vi "NIIE_ni.com_iconlibrary.vi"(8 "error in (no error)":errorcluster {"code" min=0 max=0}) -> (0 "error out":errorcluster {"code" min=0 max=0})   [LabVIEW 2021]
doc: "<p>Select <strong>Tools<span class=\"U+187\">>></span>Synchronize with ni.com Icon Library</strong> from the <a href=\"nihelplauncher://docs/csh?context=lvcore_lvdialog_icon_editor\">Icon Editor</a> dialog box to display this dialog box.</p>\n<p>Use this dialog box to synchronize the <span class=\"Monospace\">LabVIEW Data\\Glyphs</span> directory with the most recent glyphs in the <a href=\"https://www.ni.com/r/expnr7\">Icon Library</a> at <span class=\"Monospace\">ni.com</span>.</p>\n<p>This dialog box includes the following components:</p>"
uses:
  MB CORE/TypeDefs/Array_Glyph List.ctl
  MB CORE/TypeDefs/Cluster_Glyph Data.ctl
  vi.lib/LabVIEW Icon API/lv_icon/Controls/Pathes.ctl
  lv_IconEditor.lvlib
  vi.lib/LabVIEW Icon API/lv_icon/lv_icon.lvlib
panel:
  in  "Array":T1(array[cluster])
  in  "Message in":string="Downloading files..."
  in  "Abort Button Text (\"\")":string="Cancel"
  in  "FP.Title":string="Downloading Icon Library Files"
  out "Icon Library":string="Icon Library"
  in  "Select / Deselect":bool
  in  "?":T2 {"Rectangle"."left" min=0 max=0; "Rectangle"."top" min=0 max=0; "Rectangle"."right" min=0 max=0; "Rectangle"."bottom" min=0 max=0}
  out "Install":string="Install"
  out "Glyph name":string="Name"
  out "SubFolder":string="Subfolder"
  out "Current Glyph":string="Current"
  in  "Glyph list":T3=[{"Install"=FALSE, "Current"=bytes[272], "Icon Library"=bytes[272], "Subfolder"="", "Name"=""}]
  in  "Help":bool
  in  "Cancel":bool
  in  "OK":bool
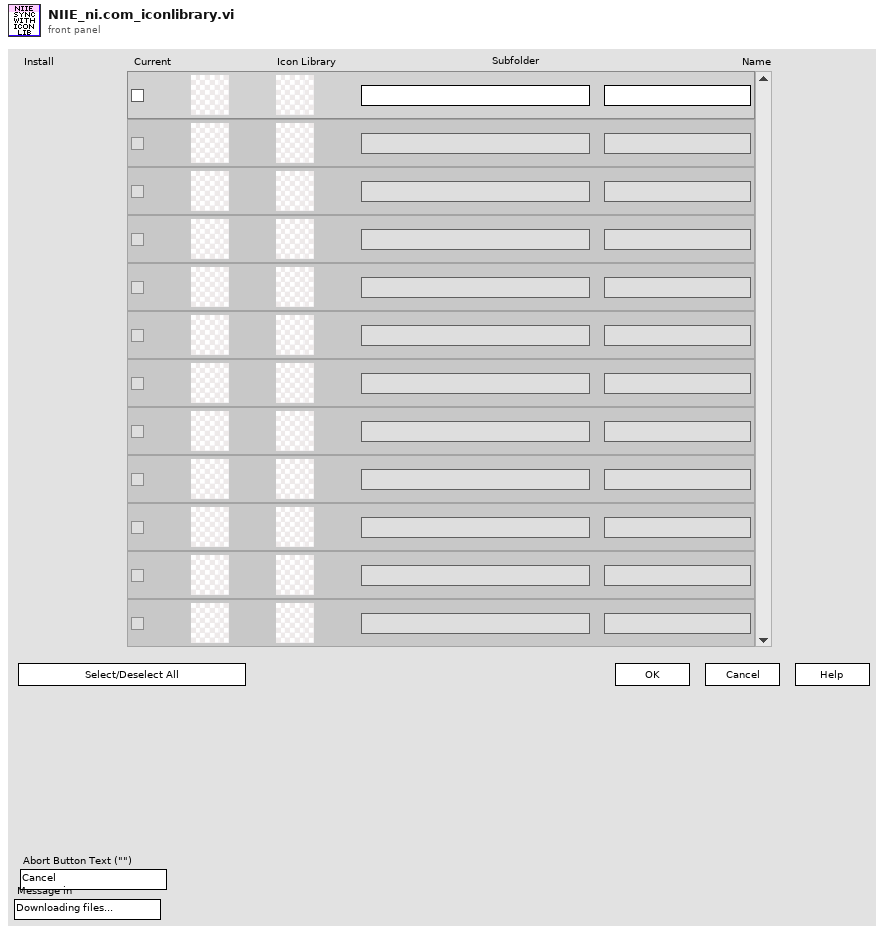
[diagram p1: front panel]
types:
  T1 = cluster{"Group folder":string, "FileName":string, "Rectangle":cluster{"left":i16, "top":i16, "right":i16, "bottom":i16}, "Path":path, "Image":picture}[]
  T2 = cluster{"Group folder":string, "FileName":string, "Rectangle":cluster{"left":i16, "top":i16, "right":i16, "bottom":i16}, "Path":path, "Image":picture}
  T3 = typedef "Array_Glyph List.ctl" = T4[]
  T4 = typedef "Cluster_Glyph Data.ctl" = cluster{"Install":bool, "Current":picture, "Icon Library":picture, "Subfolder":string, "Name":string}
  T5 = typedef "XMLDataStructureIconLibrary.ctl" = cluster{"imgExt":string, "glyphNameLoc":string, "glyphName":string, "type":string, "loctype":string, "imgName":string}
  T6 = typedef "Pathes.ctl" = enum16{"Root Path", "Icon Templates", "Icon Templates VI", "Icon Templates Lib", "Glyphs"}
  T7 = cluster{"File in zip file":string, "File name on disk":string, "Group":string}[]
  T8 = typedef "imagedata.ctl" = cluster{"image type":i32, "image depth":i32, "image":u8[], "mask":u8[], "colors":u32[], "Rectangle":cluster{"left":i16, "top":i16, "right":i16, "bottom":i16}}
  T9 = typedef "Cluster_Path&Icon.ctl" = cluster{"Rectangle":cluster{"left":i16, "top":i16, "right":i16, "bottom":i16}, "Path":path, "Image":picture, "Filter":string, "FileName":string}
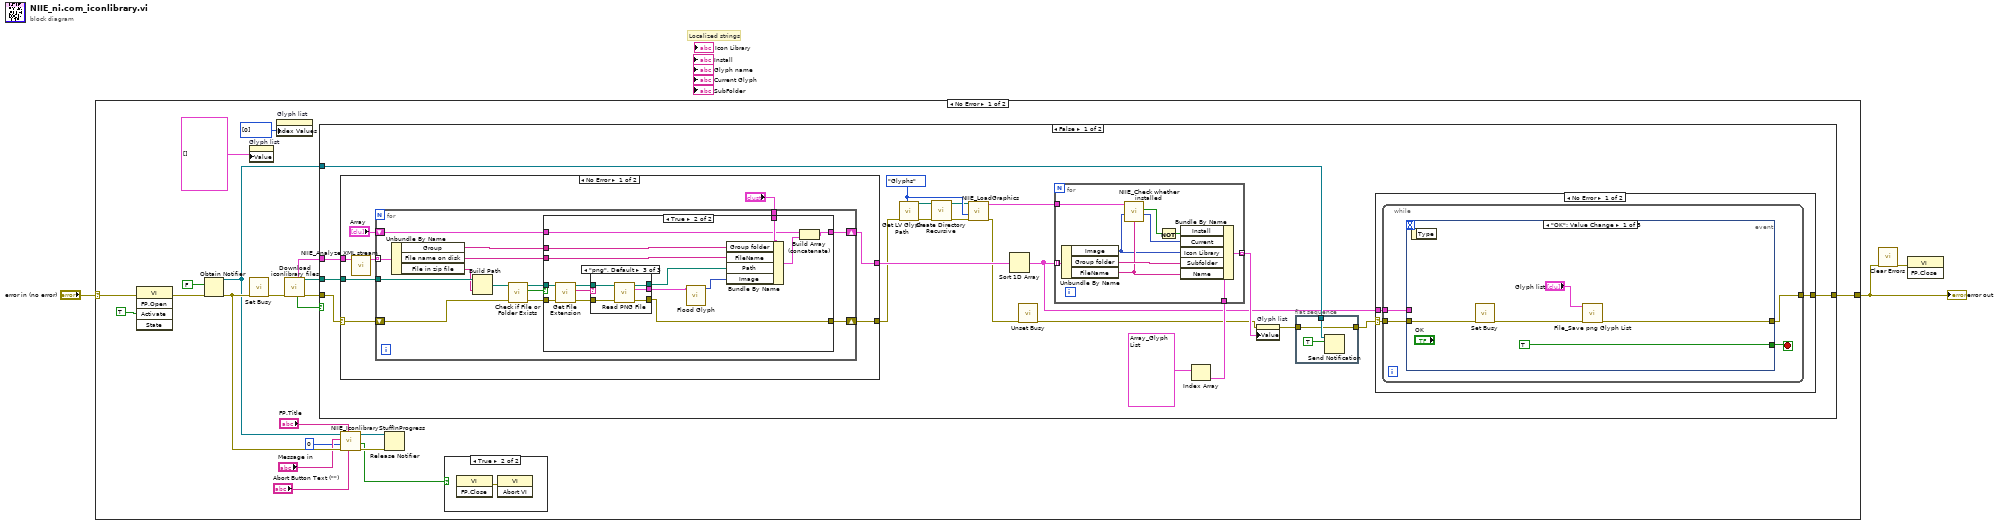
[diagram p0: block diagram]
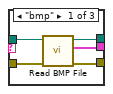
[diagram p4: hidden frame]
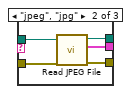
[diagram p5: hidden frame]
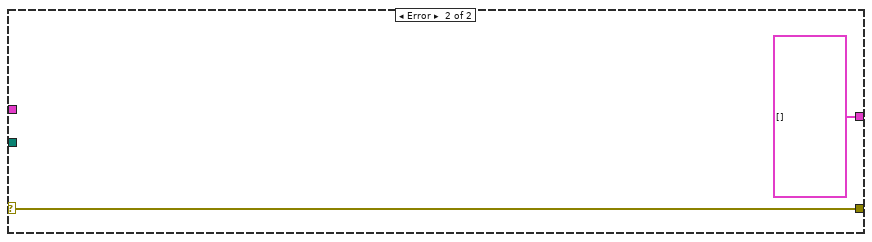
[diagram p6: hidden frame]
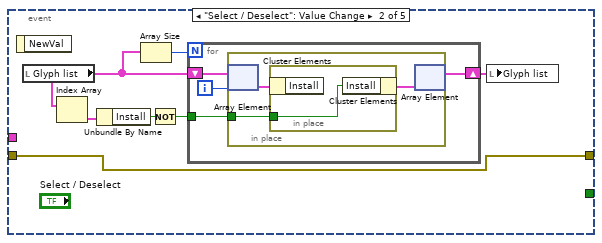
[diagram p7: hidden frame]
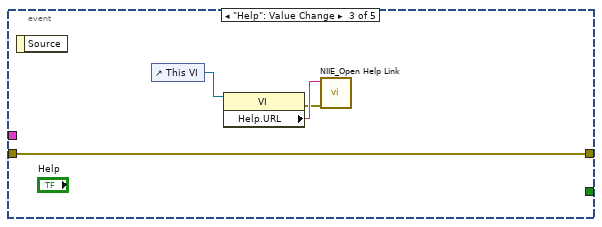
[diagram p8: hidden frame]
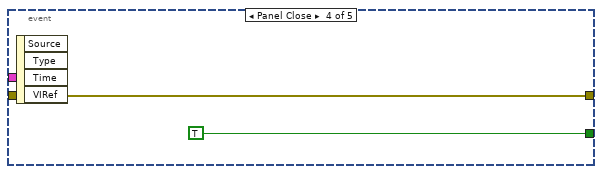
[diagram p9: hidden frame]
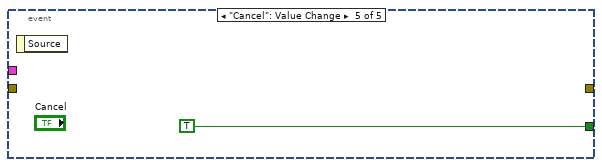
[diagram p10: hidden frame]
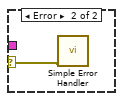
[diagram p11: hidden frame]
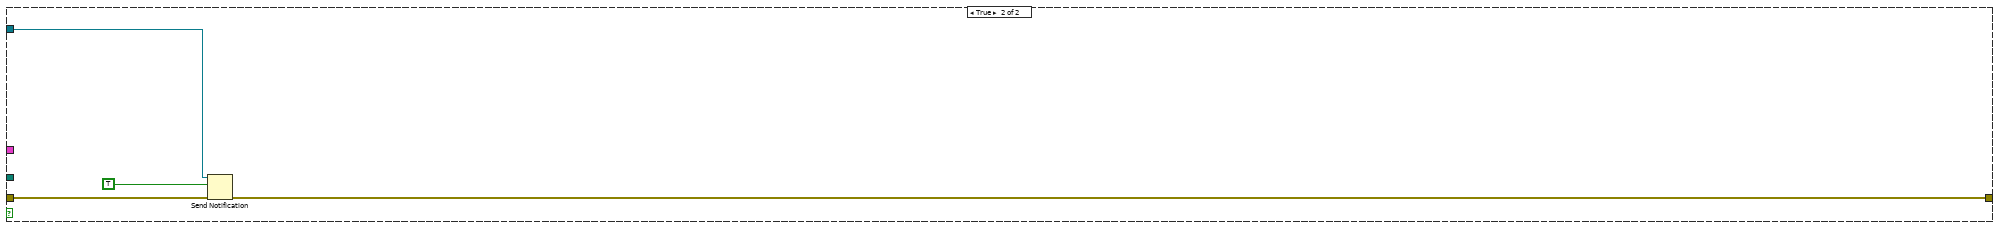
[diagram p12: hidden frame]
diagram:
  # "Localized strings"
  n1 = case shown="No Error" "error in (no error)" {
    selector: "error in (no error)" -> [w4 w155]
    tunnel: [w22 w155] -> w1
    frame No Error {
      n2 = invoke class="VI" method="FP.Open"(error in=w4, "Activate"=TRUE ("Activate?")) -> (error out=w6:errorcluster)  [unwired: 3 in, 4 out]
      n3 = Obtain Notifier(notification data type=FALSE, error in (no error)=w6) -> (notifier out=w9:refnum<notifier>, error out=w12:errorcluster)  [unwired: 2 in, 1 out]
      n4 = call <vilib>:"Set Busy.vi"("error in (no error)"=w12) -> ("error out"=w21:errorcluster)  [unwired: 3 in, 7 out]
      n5 = property on="Glyph list" class="Arr (strict)"("Value"=T3 [] ("Glyph list")) -> ()  [unwired: 2 in, 2 out]
      n6 = property on="Glyph list" class="Arr (strict)"("Index Values"=u32[] [0]) -> ()  [unwired: 2 in, 2 out]
      n7 = call "Download iconlibrary files.vi"("error in"=w21) -> ("error out"=w19:errorcluster, "parent path"=w23:path, "Cancelled?"=w17:bool, "XML Data"=w24:T5[])  [unwired: 7 out]
      n8 = case shown="False" w17 {
        tunnel: w24 -> [w46 _]
        tunnel: w23 -> [w45 _]
        tunnel: [w44 w151] -> w22
        tunnel: w19 -> [w34 w153]
        tunnel: w9 -> [w37 w152]
        frame False {
          w41 = Pathes."Glyphs" ("Path")
          n9 = case shown="No Error" w34 {
            selector: w34 -> [w49 w102]
            tunnel: w46 -> [w54 _]
            tunnel: [w48 T1 []] -> w33
            tunnel: w45 -> [w52 _]
            tunnel: [w51 w102] -> w31
            frame No Error {
              n10 = call "NIIE_Analyze XML stream.vi"("XML Data"=w54) -> ("Data"=w53:T7)  [unwired: 10 out]
              n11 = for {
                tunnel: w52 -> [w67]
                tunnel: w53 -> [w68] mode=indexing
                tunnel: "?" -> [w64]
                shift-right: [w55] -> w51
                shift-left: w49 -> [w58]
                shift-right: [w62] -> w48
                shift-left: "Array" -> [w61]
                n12 = Unbundle By Name(w68) -> ("Group"=w65:string, "File name on disk"=w63:string, "File in zip file"=w66:string)
                n13 = Build Path(base path=w67, name or relative path=w66) -> (appended path=w60:path)
                n14 = call <vilib>:"Check if File or Folder Exists.vi"("error in (no error)"=w58, "path"=w60) -> ("error out"=w56:errorcluster, "file or folder exists?"=w57:bool, "dup path"=w59:path)  [unwired: 7 in]
                n15 = case shown="True" w57 {
                  tunnel: w59 -> [_ w85]
                  tunnel: w56 -> [w69 w84]
                  tunnel: w65 -> [_ w79]
                  tunnel: w64 -> [_ w78]
                  tunnel: w63 -> [_ w77]
                  tunnel: [w70 w73] -> w62
                  tunnel: w61 -> [w70 w72]
                  tunnel: [w69 w71] -> w55
                  frame False {
                  }
                  frame True {
                    n16 = call <vilib>:"Get File Extension.vi"("error in (no error)"=w84, "file"=w85) -> ("error out"=w81:errorcluster, "lowercase file extension"=w82:string, "dup file"=w83:path)  [unwired: 7 out]
                    n17 = case shown="\"png\", Default" w82 {
                      tunnel: w83 -> [w89 w94 w100]
                      tunnel: w81 -> [w90 w95 w99]
                      tunnel: [w87 w93 w97] -> w76
                      tunnel: [w88 w92 w98] -> w80
                      tunnel: [w86 w91 w96] -> w71
                      frame "bmp" {
                        n18 = call <vilib>:"Read BMP File.vi"("error in (no error)"=w90, "path to BMP file"=w89) -> ("error out"=w86:errorcluster, "image data"=w87:T8, "path"=w88:path)  [unwired: 7 out]
                      }
                      frame "jpeg", "jpg" {
                        n19 = call <vilib>:"Read JPEG File.vi"("error in (no error)"=w95, "path to JPEG file"=w94) -> ("error out"=w91:errorcluster, "image data"=w93:T8, "path"=w92:path)  [unwired: 1 in, 6 out]
                      }
                      frame "png", Default {
                        n20 = call <vilib>:"Read PNG File.vi"("error in (no error)"=w99, "path to PNG file"=w100) -> ("error out"=w96:errorcluster, "image data"=w97:T8, "path"=w98:path)  [unwired: 1 in, 6 out]
                      }
                    }
                    n21 = call "Flood Glyph.vi"("Image Data"=w76) -> ("Pic Out"=w75:picture)  [unwired: 1 in, 9 out]
                    n22 = Bundle By Name(cluster=w78, "Group folder"=w79, "FileName"=w77, "Path"=w80, "Image"=w75) -> (w74:T2)
                    n23 = Build Array (concatenate)(w72, w74) -> (w73:T1)
                  }
                }
              }
            }
            frame Error {
            }
          }
          n24 = call "Get LV Glyph Path.vi"("Path"=w41, "error in (no error)"=w31) -> ("error out"=w30:errorcluster, "Requested Path"=w29:path)  [unwired: 1 in, 7 out]
          n25 = call <vilib>:"Create Directory Recursive.vi"("error in (no error)"=w30, "directory"=w29) -> ("error out"=w27:errorcluster, "directory copy"=w28:path)  [unwired: 1 in, 3 out]
          n26 = call "NIIE_LoadGraphics.vi"("Error"=w27, "Source"=w41, "Graphic Root Folder"=w28) -> ("Error Out"=w26:errorcluster, "Glyphs Out"=w40:T9[])  [unwired: 3 in, 4 out]
          n27 = Sort 1D Array(array=w33) -> (sorted array=w32:T1)
          n28 = call <vilib>:"Unset Busy.vi"("error in (no error)"=w26) -> ("error out"=w38:errorcluster)  [unwired: 1 in, 9 out]
          n29 = Index Array(array=T3 [{"Install"=FALSE, "Current"=bytes[272], "Icon Library"=bytes[272], "Subfolder"="", "Name"=""}] ("Cluster")) -> (element=w43:T4)  [unwired: 1 in]
          n30 = for {
            tunnel: w32 -> [w149] mode=indexing
            tunnel: w43 -> [w150]
            tunnel: w40 -> [w147]
            tunnel: [w146] -> w39 mode=indexing
            n31 = Unbundle By Name(w149) -> ("Image"=w141:picture, "Group folder"=w148:string, "FileName"=w142:string)
            n32 = call "NIIE_Check whether installed.vi"("Glyph Name"=w142, "Glyph Pic"=w141, "Glyphs[]"=w147) -> ("Image Out"=w143:picture, "Match? Out"=w145:bool)  [unwired: 1 in, 6 out]
            n33 = Not(x=w145) -> (.not. x?=w144:bool)
            n34 = Bundle By Name(cluster=w150, "Install"=w144, "Current"=w143, "Icon Library"=w141, "Subfolder"=w148, "Name"=w142) -> (w146:T4)
          }
          n35 = property on="Glyph list" class="Arr (strict)"(error in=w38, "Value"=w39) -> (error out=w36:errorcluster)  [unwired: 1 in, 1 out]
          n36 = flat-sequence {
            tunnel: w37 -> [w105]
            tunnel: w36 -> [w103]
            tunnel: [w103] -> w35
            frame #0 {
              n37 = Send Notification(notification=TRUE, notifier=w105) -> ()  [unwired: 1 in, 2 out]
            }
          }
          n38 = case shown="No Error" w35 {
            selector: w35 -> [w106 w140]
            tunnel: w32 -> [w108 _]
            tunnel: [w107 _] -> w44
            frame No Error {
              n39 = while {
                tunnel: w106 -> [w112]
                tunnel: w108 -> [w110]
                tunnel: [w109] -> w107
                stop <- w111 stop-if-true
                n40 = event shown="[0] \"OK\": Value Change" {
                  selector: _ -> [_ _ _ _ _]
                  dyn-events: _ -> [_ _ _ _ _]
                  timeout: _ -> [_ _ _ _ _]
                  tunnel: w112 -> [w115 w120 w136 w137 _]
                  tunnel: [TRUE _ _ TRUE TRUE] -> w111
                  tunnel: [w113 w120 w136 w137 _] -> w109
                  tunnel: w110 -> [_ _ _ _ _]
                  event "OK": Value Change {
                    n41 = event-data() -> ()  [unwired: 1 in, 1 out]
                    n42 = call <vilib>:"Set Busy.vi"("error in (no error)"=w115) -> ("error out"=w114:errorcluster)  [unwired: 3 in, 7 out]
                    n43 = call "File_Save png Glyph List.vi"("error in (no error)"=w114, "Glyph list"="Glyph list") -> ("error out"=w113:errorcluster)  [unwired: 9 out]
                  }
                  event "Select / Deselect": Value Change {
                    n44 = event-data() -> ()  [unwired: 1 in, 1 out]
                    n45 = local read "Glyph list"() -> (w118:T3)
                    n46 = Index Array(array=w118) -> (element=w124:T4)  [unwired: 1 in]
                    n47 = Unbundle By Name(w124) -> ("Install"=w123:bool)
                    n48 = Array Size(array=w118) -> (size(s)=w119:i32)
                    n49 = Not(x=w123) -> (.not. x?=w122:bool)
                    n50 = for {
                      N: w119 -> [_]
                      shift-right: [w125] -> w121
                      shift-left: w118 -> [w128]
                      tunnel: w122 -> [w126]
                      i -> [w127]
                      n51 = in-place {
                        in-place-border: w126 -> [w130]
                        n52 = in-place-array #1(w128, w127) -> (w131:T4)
                        n53 = in-place {
                          in-place-border: w130 -> [w132]
                          n54 = in-place-cluster #2(w131) -> ()  [unwired: 1 out]
                          n55 = in-place-cluster #2("Install"=w132) -> (w129:T4)
                        }
                        n56 = in-place-array #1(w129) -> (w125:T3)  [unwired: 1 out]
                      }
                    }
                    n57 = local write "Glyph list"(w121) -> ()
                  }
                  event "Help": Value Change {
                    n58 = event-data() -> ()  [unwired: 1 in, 1 out]
                    n59 = control-ref of="This VI"() -> (w135:refnum<vi>)
                    n60 = property class="VI"(reference=w135) -> (error out=w133:errorcluster, "Help.URL"=w134:string)  [unwired: 1 in, 1 out]
                    n61 = call "NIIE_Open Help Link.vi"("error in (no error)"=w133, "Help.URL"=w134) -> ()  [unwired: 9 in, 1 out]
                  }
                  event Panel Close {
                    n62 = event-data() -> ()  [unwired: 1 in, 4 out]
                  }
                  event "Cancel": Value Change {
                    n63 = event-data() -> ()  [unwired: 1 in, 1 out]
                  }
                }
              }
            }
            frame Error {
              n64 = call <vilib>:"Simple Error Handler.vi"("error in (no error)"=w140) -> ()  [unwired: 3 in, 6 out]
            }
          }
        }
        frame True {
          n65 = Send Notification(notification=TRUE, notifier=w152, error in (no error)=w153) -> (error out=w151:errorcluster)  [unwired: 1 out]
        }
      }
      n66 = call "NIIE_IconlibraryStuffInProgress.vi"("Abort Button Text (\"\")"="Abort Button Text (\"\")", "FP.Title"="FP.Title", "error in (no error)"=w12, "Show FP Timeout (ms)"=0, "Message in"="Message in", "Close Notifier"=w9) -> ("error out"=w15:errorcluster, "Aborted"=w10:bool, "Close Notifier out"=w14:refnum<notifier>)  [unwired: 3 in]
      n67 = Release Notifier(notifier=w14, error in (no error)=w15) -> ()  [unwired: 1 in, 3 out]
      n68 = case shown="True" w10 {
        frame False {
        }
        frame True {
          n69 = invoke class="VI" method="FP.Close"() -> (error out=w25:errorcluster)  [unwired: 3 in, 2 out]
          n70 = invoke class="VI" method="Abort VI"(error in=w25) -> ()  [unwired: 2 in, 3 out]
        }
      }
    }
    frame Error {
    }
  }
  "error out" <- w1
  n71 = call <vilib>:"Clear Errors.vi"("error in (no error)"=w1) -> ("error out"=w2:errorcluster)  [unwired: 5 in, 1 out]
  n72 = invoke class="VI" method="FP.Close"(error in=w2) -> ()  [unwired: 2 in, 3 out]
